vi "Agilent_Init_Array.vi"(1 "Agilent Array In":T1[](array[typedef])) -> (0 "Agilent Array Out":T1[](array[typedef]))   [LabVIEW 2020]
uses:
  AgilentTotalCluster.ctl
  AgilentControl.ctl
  Channel Config.ctl
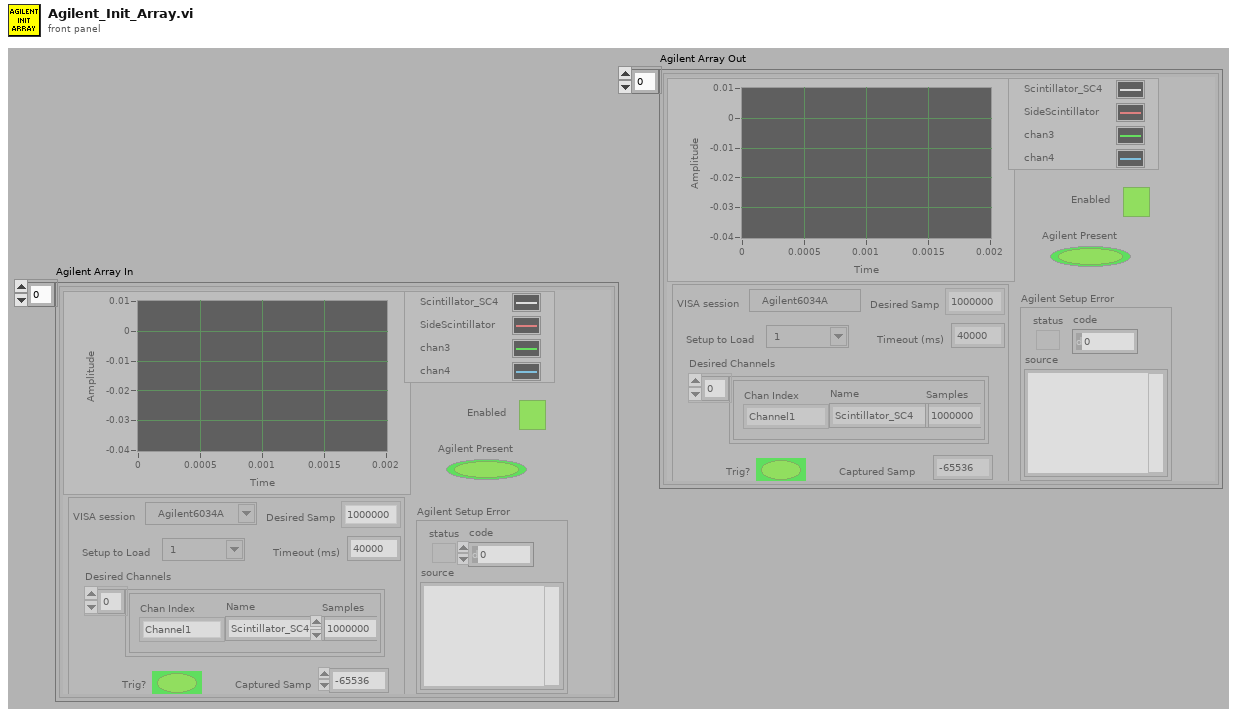
[diagram p1: front panel]
types:
  T1 = typedef "AgilentTotalCluster.ctl" = cluster{"Agilent Graph":waveform(dbl)[], "Agilent Control":T2, "Agilent Setup Error":errorcluster, "Agilent Present":bool, "Enabled":bool}
  T2 = typedef "AgilentControl.ctl" = cluster{"Trig?":bool, "VISA session":refnum<visa-resource-name>, "Setup to Load":string, "Timeout (ms)":u32, "Desired Samp":enum32{"100", "250", "500", "1000", "2000", "5000", "10000", "20000", "50000", "100000", "200000", "500000", "1000000", "2000000", "4000000", "8000000"}, "Captured Samp":i32, "Desired Channels":T3[]}
  T3 = typedef "Channel Config.ctl" = cluster{"Chan Index":enum16{"Channel1", "Channel2", "Channel3", "Channel4", "MATH"}, "Name":string, "Samples":i32}
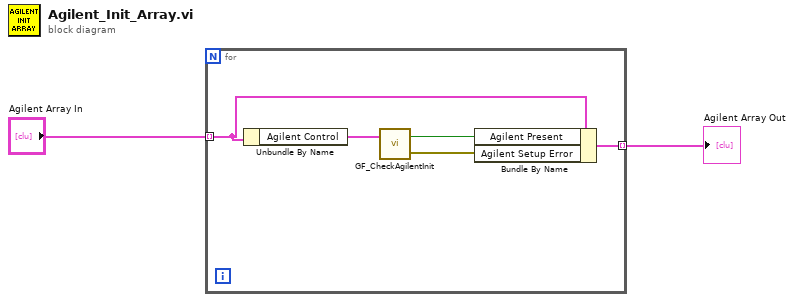
[diagram p0: block diagram]
diagram:
  n1 = for {
    tunnel: "Agilent Array In" -> [w6] mode=indexing
    tunnel: [w3] -> w1 mode=indexing
    n2 = Unbundle By Name(w6) -> ("Agilent Control"=w7:T2)
    n3 = call "GF_CheckAgilentInit.vi"("Agilent Control In"=w7) -> ("Success"=w4:bool, "error out"=w5:errorcluster)
    n4 = Bundle By Name(cluster=w6, "Agilent Present"=w4, "Agilent Setup Error"=w5) -> (w3:T1)
  }
  "Agilent Array Out" <- w1
